vi "StdDeviation.vi"(11 "2D  Array":u64[][](array[numeric]) format="%.1f") -> (0 "Deviation by row":i64[][](array[numeric]) format="%.1f", 1 "STD":dbl[](array[numeric]), 2 "Variance":dbl[](array[numeric]), 3 "Average in row":u64[](array[numeric]) format="%-2.0f")   [LabVIEW 2023]
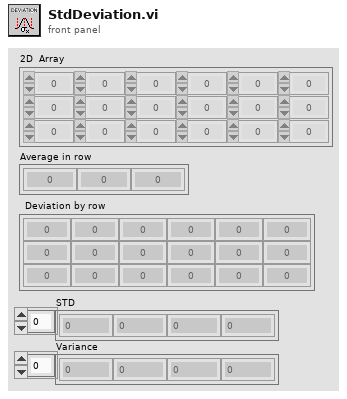
[diagram p1: front panel]
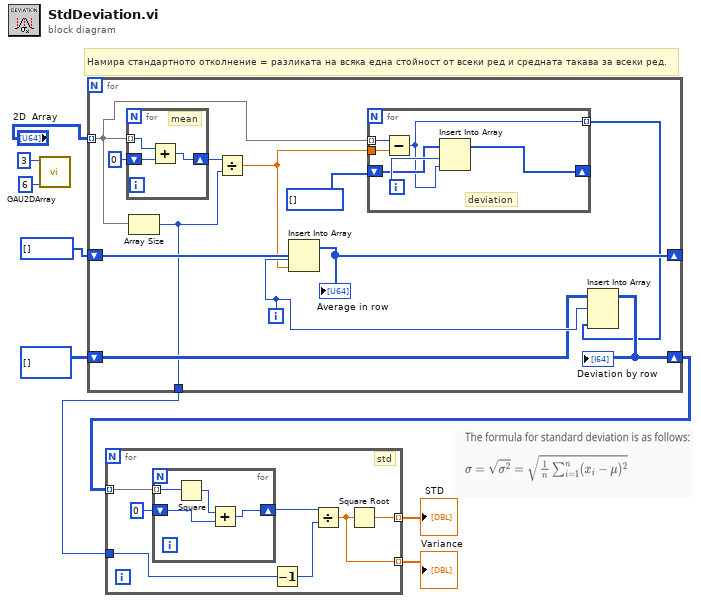
[diagram p0: block diagram]
diagram:
  # "Намира стандартното отколнение = разликата на всяка една стойност от всеки ред и средната такава за всеки ред."
  n1 = call "GAU2DArray.vi"("Colums"=6, "Rows"=3) -> ()  [unwired: 8 in, 2 out]
  n2 = for {
    tunnel: "2D  Array" -> [w12] mode=indexing
    shift-right: [w17] -> _
    shift-left: u64[] [] -> [w20]
    shift-right: [w14] -> w4
    shift-left: i64[][] [] -> [w15]
    tunnel: [w10] -> w1
    i -> [w16]
    n3 = for {
      tunnel: w12 -> [w30] mode=indexing
      shift-right: [w29] -> w19
      shift-left: 0 -> [w28]
      # "mean"
      n4 = Add(x=w30, y=w28) -> (x+y=w29:u64)
    }
    n5 = Array Size(array=w12) -> (size(s)=w10:i32)
    n6 = Divide(x=w19, y=w10) -> (x/y=w13:dbl)
    n7 = Insert Into Array "Insert Into Array"(array=w20, index=w16, new element=w13) -> (w17:u64[])
    "Average in row" <- w17
    n8 = for {
      tunnel: w12 -> [w27] mode=indexing
      tunnel: w13 -> [w26]
      shift-right: [w23] -> _
      shift-left: u64[] [] -> [w24]
      tunnel: [w22] -> w11 mode=indexing
      i -> [w25]
      # "deviation"
      n9 = Subtract(x=w27, y=w26) -> (x-y=w22:i64)
      n10 = Insert Into Array "Insert Into Array"(array=w24, index=w25, new element=w22) -> (w23:u64[])
    }
    n11 = Insert Into Array "Insert Into Array"(array=w15, index (row)=w16, new element=w11) -> (w14:i64[][])  [unwired: 1 in]
    "Deviation by row" <- w14
  }
  n12 = for {
    tunnel: w4 -> [w37] mode=indexing
    tunnel: [w34] -> w3 mode=indexing
    tunnel: [w33] -> w2 mode=indexing
    tunnel: w1 -> [w32]
    # "std"
    n13 = for {
      tunnel: w37 -> [w41] mode=indexing
      shift-right: [w39] -> w35
      shift-left: i64 0 -> [w38]
      n14 = Square(x=w41) -> (x^2=w40:i64)
      n15 = Add(x=w40, y=w38) -> (x+y=w39:i64)
    }
    n16 = Decrement(x=w32) -> (x-1=w31:i32)
    n17 = Divide(x=w35, y=w31) -> (x/y=w33:dbl)
    n18 = Square Root(x=w33) -> (sqrt(x)=w34:dbl)
  }
  "STD" <- w3
  "Variance" <- w2
